vi "CC Launch Object.vi"(7 "Config File Path":path, 8 "error in (no error)":errorcluster, 9 "Path to Instruments":path, 10 "system settings":T1, 11 "Inst Model":string) -> (0 "error out":errorcluster, 2 "vi ref":refnum<vi>, 3 "VI Clone Name":string)   [LabVIEW 2019]
uses:
  SS typedef cluster Instrument Cmd Q Init Parameters.ctl
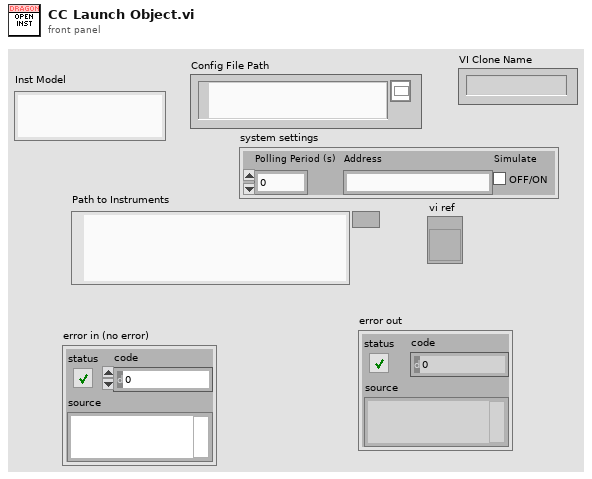
[diagram p1: front panel]
types:
  T1 = typedef "SS typedef cluster Instrument Cmd Q Init Parameters.ctl" = cluster{"Polling Period (s)":dbl, "Address":string, "Simulate":bool}
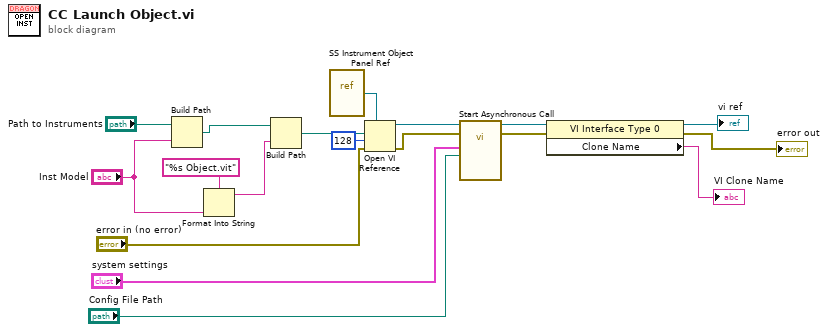
[diagram p0: block diagram]
diagram:
  n1 = Build Path(base path="Path to Instruments", name or relative path="Inst Model") -> (appended path=w17:path)
  n2 = Format Into String(format string="%s Object.vit", "Inst Model") -> (resulting string=w16:string)  [unwired: 2 in, 1 out]
  n3 = Build Path(base path=w17, name or relative path=w16) -> (appended path=w2:path)
  n4 = vi-ref "SS Instrument Object Panel Ref.vi"() -> (w15:refnum<vi>)
  n5 = Open VI Reference(type specifier VI Refnum (for type only)=w15, vi path=w2, options=128, error in (no error)="error in (no error)") -> (vi reference=w8:refnum<vi>, error out=w7:errorcluster)  [unwired: 2 in]
  n6 = call-by-ref "Start Asynchronous Call"(reference=w8, error in=w7, "Config File Path"="Config File Path", "system settings"="system settings") -> (reference out=w6:refnum<vi>, error out=w4:errorcluster)  [unwired: 9 in, 1 out]
  n7 = property class="VI Interface Type 0"(reference=w6, error in=w4) -> (reference out=→"vi ref":refnum<vi>, error out=→"error out":errorcluster, "Clone Name"=→"VI Clone Name":string)
